vi "Handshake.vi"(8 "error in (no error)":errorcluster, 9 "timeout in ms (10000)":i32=10000, 11 "Local Queues in":T1) -> (0 "error out":errorcluster, 3 "Local Queues out":T1)   [LabVIEW 2020, in "Communication VIs.lvlib" / "Local.lvlib"]
uses:
  Local.lvlib
  Local Queues.ctl
  <vilib>/Utility/error.llb/Error Cluster From Error Code.vi
  <vilib>/ErrorRing/Error Ring.xnode
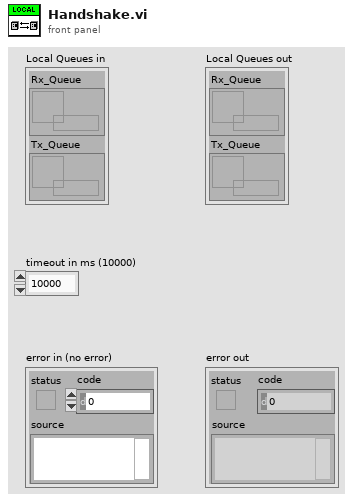
[diagram p1: front panel]
types:
  T1 = typedef "Communication VIs.lvlib/Local.lvlib/Local Queues.ctl" = cluster{"Rx_Queue":refnum<queue>, "Tx_Queue":refnum<queue>}
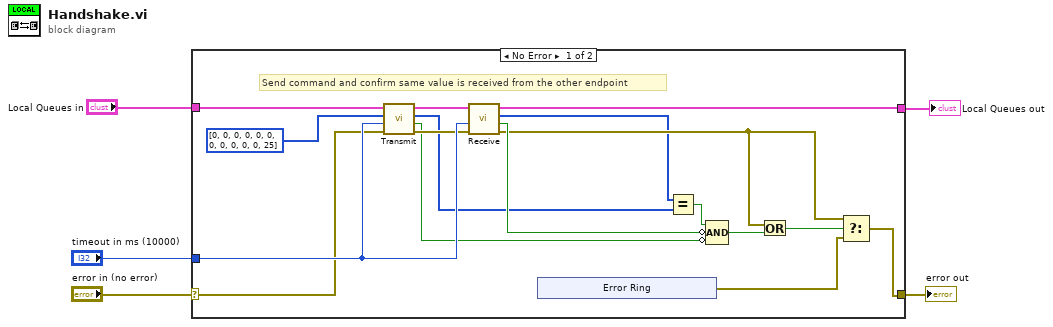
[diagram p0: block diagram]
diagram:
  n1 = case shown="No Error" "error in (no error)" {
    selector: "error in (no error)" -> [w7 w29]
    tunnel: [w18 w29] -> w4
    tunnel: [w11 w28] -> w1
    tunnel: "Local Queues in" -> [w22 w28]
    tunnel: "timeout in ms (10000)" -> [w21 _]
    frame No Error {
      # "Send command and confirm same value is received from the other endpoint"
      n2 = call "Transmit.vi"("error in (no error)"=w7, "timeout in ms (-1)"=w21, "Packet Data"=u8[] [0, 0, 0, 0, 0, 0, 0, 0, 0, 0, 0, 25], "Local Queues in"=w22) -> ("error out"=w20:errorcluster, "Timeout?"=w16:bool, "Packet Data Sent"=w6:u8[], "Local Queues out"=w12:T1)  [unwired: 4 in]
      n3 = call "Receive.vi"("error in (no error)"=w20, "timeout in ms (0)"=w21, "Local Queues in"=w12) -> ("error out"=w10:errorcluster, "Timeout?"=w17:bool, "Packet Received"=w9:u8[], "Local Queues out"=w11:T1)  [unwired: 5 in]
      n4 = xnode "Error Ring"() -> ("error out"=w19:errorcluster)
      n5 = Equal?(x=w9, y=w6) -> (x = y?=w15:bool)
      n6 = Compound Arithmetic op=AND(w15, invert w17, invert w16) -> (w14:bool)
      n7 = Or(x=w10, y=w14) -> (x .or. y?=w13:bool)
      n8 = Select(t=w10, s=w13, f=w19) -> (s? t:f=w18:errorcluster)
    }
    frame Error {
    }
  }
  "error out" <- w4
  "Local Queues out" <- w1
